vi "Read PV Monitor Actor's Enqueuers.vi"(8 "error in (no error)":errorcluster, 11 "CS++ControllerActor in":refnum<class "CS++PVProxy.lvclass">) -> (0 "error out":errorcluster, 2 "PV Monitor Actor's Enqueuers":refnum<class "Message Enqueuer.lvclass">[](array[class]), 3 "CS++ControllerActor out":refnum<class "CS++PVProxy.lvclass">)   [LabVIEW 2014, in "CS++PVProxy.lvlib" / "CS++PVProxy.lvclass"]
uses:
  CS++PVProxy.lvclass
  <vilib>/ActorFramework/Message Enqueuer/Message Enqueuer.lvclass
  CS++PVProxy.lvclass/CS++PVProxy.ctl
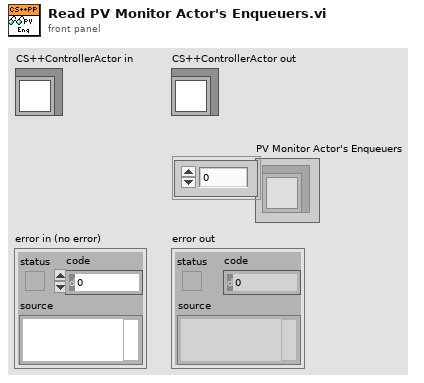
[diagram p1: front panel]
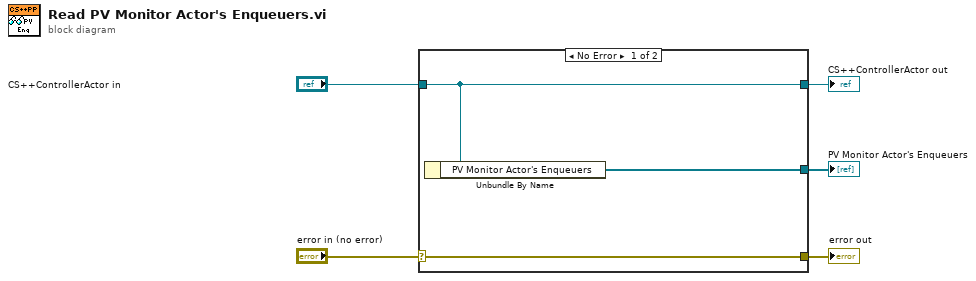
[diagram p0: block diagram]
diagram:
  n1 = case shown="No Error" "error in (no error)" {
    selector: "error in (no error)" -> [w8 w9]
    tunnel: [w8 w9] -> w4
    tunnel: [w7 w10] -> w2
    tunnel: "CS++ControllerActor in" -> [w7 w10]
    tunnel: [w6 _] -> w1
    frame No Error {
      n2 = Unbundle By Name(w7) -> ("PV Monitor Actor's Enqueuers"=w6:refnum<class "Message Enqueuer.lvclass">[])
    }
    frame Error {
    }
  }
  "error out" <- w4
  "CS++ControllerActor out" <- w2
  "PV Monitor Actor's Enqueuers" <- w1
